vi "IMU read.vi"(8 "error in (no error)":errorcluster, 11 "Refnum in":T1) -> (0 "error out":errorcluster, 1 "g-x":dbl, 2 "a-z":dbl, 3 "Refnum out":T1, 4 "g-z":dbl, 5 "a-y":dbl, 6 "g-y":dbl, 7 "a-x":dbl)   [LabVIEW 2014]
uses:
  LabView/roger-i2c/Host API/Controls/FPGA I2C_FPGA Ref.ctl
  LabView/roger-i2c/Host API/I2C Host API.lvlib
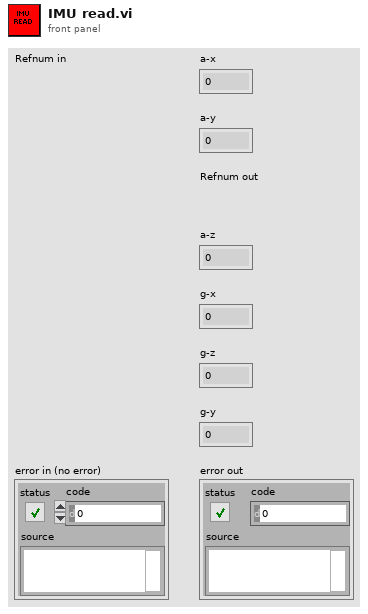
[diagram p1: front panel]
types:
  T1 = typedef "FPGA I2C_FPGA Ref.ctl" = refnum<k20>
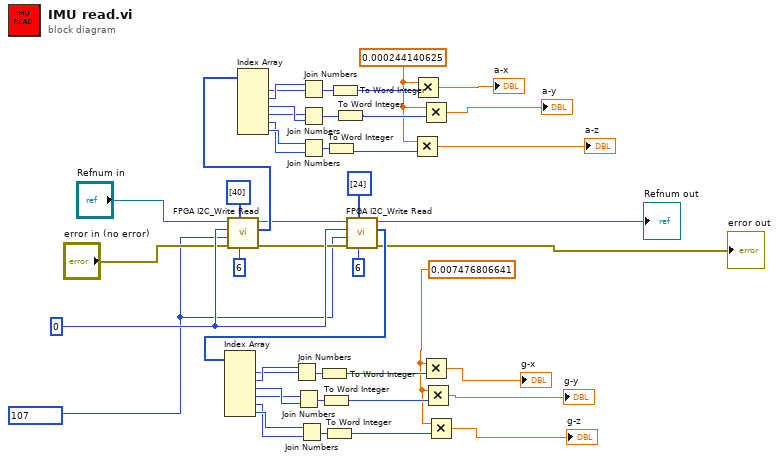
[diagram p0: block diagram]
diagram:
  w1 = u16 107 ("I2C_Address")
  w10 = u8 0 ("Port")
  w40 = 0.007476806641 ("x")
  w33 = 0.000244140625 ("x")
  n1 = call "FPGA I2C_Write Read.vi"("Bytes To Read"=u16 6 ("byte da leggere 2"), "Write Data"=u8[] [40] ("registro da leggere 2"), "error in"="error in (no error)", "I2C_Address"=w1, "Port"=w10, "FPGA VI Reference"="Refnum in") -> ("error out"=w9:errorcluster, "Read Data"=w13:u8[], "FPGA VI Reference Out"=w8:T1)  [unwired: 3 out]
  n2 = Index Array(array=w13) -> (element #1=w15:u8, element #2=w16:u8, element #3=w19:u8, element #4=w18:u8, element #5=w20:u8, element #6=w21:u8)  [unwired: 6 in]
  n3 = Join Numbers(hi=w16, lo=w15) -> ((hi.lo)=w14:u16)
  n4 = Join Numbers(hi=w18, lo=w19) -> ((hi.lo)=w17:u16)
  n5 = Join Numbers(hi=w21, lo=w20) -> ((hi.lo)=w32:u16)
  n6 = To Word Integer(number=w32) -> (16bit integer=w36:i16)
  n7 = To Word Integer(number=w14) -> (16bit integer=w35:i16)
  n8 = To Word Integer(number=w17) -> (16bit integer=w34:i16)
  n9 = call "FPGA I2C_Write Read.vi"("Bytes To Read"=u16 6 ("byte da leggere 2"), "Write Data"=u8[] [24] ("registro da leggere 2"), "error in"=w9, "I2C_Address"=w1, "Port"=w10, "FPGA VI Reference"=w8) -> ("error out"=→"error out":errorcluster, "Read Data"=w31:u8[], "FPGA VI Reference Out"=→"Refnum out":T1)  [unwired: 3 out]
  n10 = Index Array(array=w31) -> (element #1=w23:u8, element #2=w24:u8, element #3=w28:u8, element #4=w27:u8, element #5=w29:u8, element #6=w30:u8)  [unwired: 6 in]
  n11 = Join Numbers(hi=w24, lo=w23) -> ((hi.lo)=w22:u16)
  n12 = Join Numbers(hi=w27, lo=w28) -> ((hi.lo)=w25:u16)
  n13 = Join Numbers(hi=w30, lo=w29) -> ((hi.lo)=w26:u16)
  n14 = To Word Integer(number=w22) -> (16bit integer=w41:i16)
  n15 = To Word Integer(number=w25) -> (16bit integer=w42:i16)
  n16 = To Word Integer(number=w26) -> (16bit integer=w43:i16)
  n17 = Multiply(x=w33, y=w36) -> (x*y=→"a-z":dbl)
  n18 = Multiply(x=w33, y=w35) -> (x*y=→"a-x":dbl)
  n19 = Multiply(x=w33, y=w34) -> (x*y=→"a-y":dbl)
  n20 = Multiply(x=w40, y=w41) -> (x*y=→"g-x":dbl)
  n21 = Multiply(x=w40, y=w42) -> (x*y=→"g-y":dbl)
  n22 = Multiply(x=w40, y=w43) -> (x*y=→"g-z":dbl)
